vi "Periodic Tasks.vi"(8 "error in":errorcluster) -> ()   [LabVIEW 2020]
doc: "This VI runs in parallel to other tasks. It can contain as many user-defined periodic loops as you need. These can carry out PID or other sorts of timed response."
uses:
  <vilib>/Rock Robotics/WPI/Utilities/WPI_GetSetVariantRefNum.vi
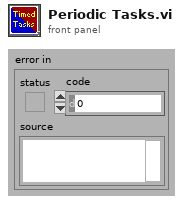
[diagram p1: front panel]
types:
  T1 = typedef "WPI_MotorControlDeviceRef.ctl" = cluster{"DeviceStatus":errorcluster, "Type":T2, "PWM":cluster{"PWM Channel":T3, "DeadBand":T4}, "CAN":cluster{"Device Number":u8, "SetOutput VI Ref":variant, "GetOutput VI Ref":variant, "Enable VI Ref":variant, "Disable VI Ref":variant, "Data":variant}, "Invert":bool, "DIO PWM":cluster{"PWM \"Enable\" Channel":T3, "DIOChannel":T5, "PWM Rate":dbl}}
  T2 = typedef "WPI_MotorControlType.ctl" = enum16{"PWM", "CAN", "DIO PWM"}
  T3 = typedef "FPGA_DIOPWMChannel.ctl" = enum8{"PWM 0", "PWM 1", "PWM 2", "PWM 3", "PWM 4", "PWM 5", "PWM 6", "PWM 7", "PWM 8", "PWM 9", "PWM MXP 0", "PWM MXP 1", "PWM MXP 2", "PWM MXP 3", "PWM MXP 4", "PWM MXP 5", "PWM MXP 6", "PWM MXP 7", "PWM MXP 8", "PWM MXP 9", "Invalid"}
  T4 = typedef "WPI_PWMDeadband.ctl" = cluster{"Name":string, "maxPositivePwm":i32, "minPositivePwm":i32, "centerPwm":i32, "maxNegativePwm":i32, "minNegativePwm":i32, "angularRange":u16}
  T5 = typedef "FPGA_DIOChannel.ctl" = enum8{"DIO 0", "DIO 1", "DIO 2", "DIO 3", "DIO 4", "DIO 5", "DIO 6", "DIO 7", "DIO 8", "DIO 9", "DIO MXP 0", "DIO MXP 1", "DIO MXP 2", "DIO MXP 3", "DIO MXP 4", "DIO MXP 5", "DIO MXP 6", "DIO MXP 7", "DIO MXP 8", "DIO MXP 9", "DIO MXP 10", "DIO MXP 11", "DIO MXP 12", "DIO MXP 13", "DIO MXP 14", "DIO MXP 15", "SPI Port CS1", "SPI Port CS2", "SPI Port CS3", "SPI Port MISO", "SPI Port MOSI", "Invalid"}
  T6 = typedef "WPI_RobotDriveDevRef.ctl" = cluster{"DevStatus":errorcluster, "Motors[]":T1[], "Square Inputs":bool, "Max Output":dbl}
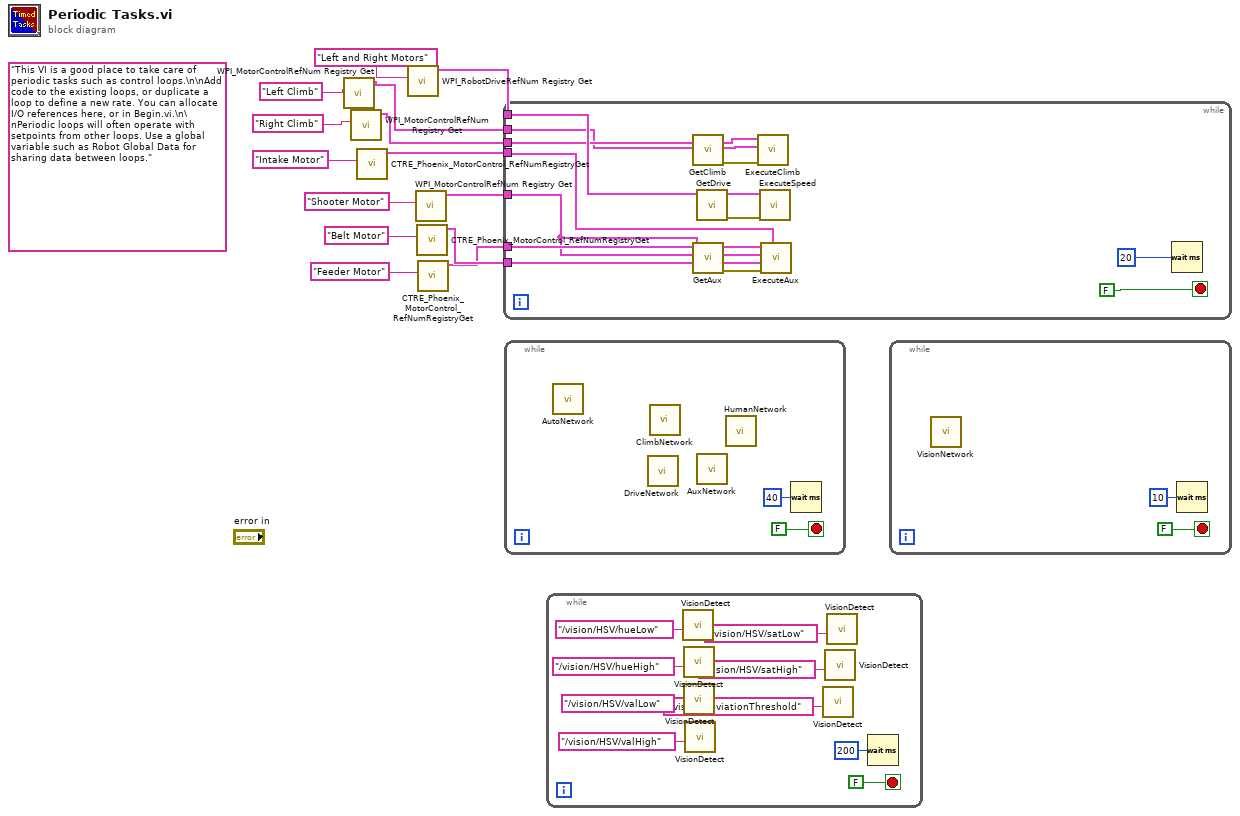
[diagram p0: block diagram]
diagram:
  (unwired) "This VI is a good place to take care of periodic tasks such as control loops.\n\nAdd code to the existing loops, or duplicate a loop to define a new rate. You can allocate I/O references here, or in Begin.vi.\n\nPeriodic loops will often operate with setpoints from other loops. Use a global variable such as Robot Global Data for sharing data between loops."
  n1 = call <vilib>:"WPI_MotorControlRefNum Registry Get.vi"("refnum name"="Left Climb") -> ("MotorControlDevRef"=w4:T1)  [unwired: 9 in, 1 out]
  n2 = call <vilib>:"WPI_MotorControlRefNum Registry Get.vi"("refnum name"="Right Climb") -> ("MotorControlDevRef"=w1:T1)  [unwired: 9 in, 1 out]
  n3 = call <vilib>:"CTRE_Phoenix_MotorControl_RefNumRegistryGet.vi"("refnum name"="Intake Motor") -> ("PhoenixMotorControlDevRef"=w7:T1)  [unwired: 9 in, 1 out]
  n4 = call <vilib>:"WPI_RobotDriveRefNum Registry Get.vi"("refnum name"="Left and Right Motors") -> ("RobotDriveDevRef"=w13:T6)  [unwired: 1 in, 9 out]
  n5 = call <vilib>:"WPI_MotorControlRefNum Registry Get.vi"("refnum name"="Shooter Motor") -> ("MotorControlDevRef"=w6:T1)  [unwired: 9 in, 1 out]
  n6 = call <vilib>:"CTRE_Phoenix_MotorControl_RefNumRegistryGet.vi"("refnum name"="Belt Motor") -> ("PhoenixMotorControlDevRef"=w10:T1)  [unwired: 9 in, 1 out]
  n7 = call <vilib>:"CTRE_Phoenix_MotorControl_RefNumRegistryGet.vi"("refnum name"="Feeder Motor") -> ("PhoenixMotorControlDevRef"=w9:T1)  [unwired: 9 in, 1 out]
  n8 = while {
    tunnel: w13 -> [w24]
    tunnel: w6 -> [w15]
    tunnel: w10 -> [w23]
    tunnel: w9 -> [w22]
    tunnel: w7 -> [w21]
    tunnel: w1 -> [w18]
    tunnel: w4 -> [w17]
    stop <- FALSE stop-if-true
    n9 = call "GetClimb.vi"() -> ("Error Out"=w16:errorcluster)  [unwired: 11 in]
    n10 = call "GetAux.vi"("Shooter Motor"=w15) -> ("Error Out"=w19:errorcluster)  [unwired: 10 in]
    n11 = call "GetDrive.vi"() -> ("Error Out"=w20:errorcluster)  [unwired: 11 in]
    n12 = call "ExecuteClimb.vi"("Error In"=w16, "Left Climb"=w17, "Right Climb"=w18) -> ()  [unwired: 8 in, 1 out]
    n13 = call "ExecuteSpeed.vi"("Error In"=w20, "RobotDriveDevRef"=w24) -> ()  [unwired: 9 in, 1 out]
    n14 = call "ExecuteAux.vi"("Intake Motor"=w21, "error in"=w19, "Belt Motor"=w23, "Shooter Motor"=w15, "Feeder Motor"=w22) -> ()  [unwired: 6 in, 1 out]
    n15 = Wait (ms)(milliseconds to wait=u32 20) -> ()  [unwired: 1 out]
  }
  n16 = while {
    stop <- FALSE stop-if-true
    n17 = call "AutoNetwork.vi"() -> ()  [unwired: 12 in]
    n18 = call "DriveNetwork.vi"() -> ()  [unwired: 12 in]
    n19 = call "ClimbNetwork.vi"() -> ()  [unwired: 12 in]
    n20 = call "AuxNetwork.vi"() -> ()  [unwired: 12 in]
    n21 = call "HumanNetwork.vi"() -> ()  [unwired: 12 in]
    n22 = Wait (ms)(milliseconds to wait=u32 40) -> ()  [unwired: 1 out]
  }
  n23 = while {
    stop <- FALSE stop-if-true
    n24 = call "VisionDetect.vi"("Name"="/vision/HSV/hueLow") -> ()  [unwired: 11 in]
    n25 = call "VisionDetect.vi"("Name"="/vision/HSV/hueHigh") -> ()  [unwired: 11 in]
    n26 = call "VisionDetect.vi"("Name"="/vision/HSV/valLow") -> ()  [unwired: 11 in]
    n27 = call "VisionDetect.vi"("Name"="/vision/HSV/valHigh") -> ()  [unwired: 11 in]
    n28 = call "VisionDetect.vi"("Name"="/vision/deviationThreshold") -> ()  [unwired: 11 in]
    n29 = call "VisionDetect.vi"("Name"="/vision/HSV/satHigh") -> ()  [unwired: 11 in]
    n30 = call "VisionDetect.vi"("Name"="/vision/HSV/satLow") -> ()  [unwired: 11 in]
    n31 = Wait (ms)(milliseconds to wait=u32 200) -> ()  [unwired: 1 out]
  }
  n32 = while {
    stop <- FALSE stop-if-true
    n33 = call "VisionNetwork.vi"() -> ()  [unwired: 12 in]
    n34 = Wait (ms)(milliseconds to wait=u32 10) -> ()  [unwired: 1 out]
  }
